vi "Test adler32.vi"() -> (3 "All Passed?":bool)   [LabVIEW 2022 SP3]
uses:
  Source/LabVIEW-Hashlib.lvlib
panel:
  out "ADLER-32 out":T1(array[cluster]) {"ADLER-32" format="%08x"}
  in  "ADLER-32 Tests":T2(array[cluster])=[{"Name"="ADLER-32/Empty", "ADLER-32"=1, "Data"="", "Initial"=1}, {"Name"="ADLER-32/Short", "ADLER-32"=300286872, "Data"="Wikipedia", "Initial"=1}, {"Name"="ADLER-32/Long", "ADLER-32"=159591549, "Data"="abcdefghijklmnopqrstuvwxyzabcdefghijklmnopqrstuvwxyzabcdefghijklmnopqrstuvwxyzabcdefghijklmnopqrstuvwxyz", "Initial"=1}, {"Name"="ADLER-32/Concat", "ADLER-32"=645159161, "Data"="abcdefghijklmnopqrstuvwxyzabcdefghijklmnopqrstuvwxyzabcdefghijklmnopqrstuvwxyzabcdefghijklmnopqrstuvwxyz", "Initial"=159591549}] {"ADLER-32" format="%08x"; "Initial" format="%08x"}
  # "http://www.unit-conversion.info/texttools/adler-32/"
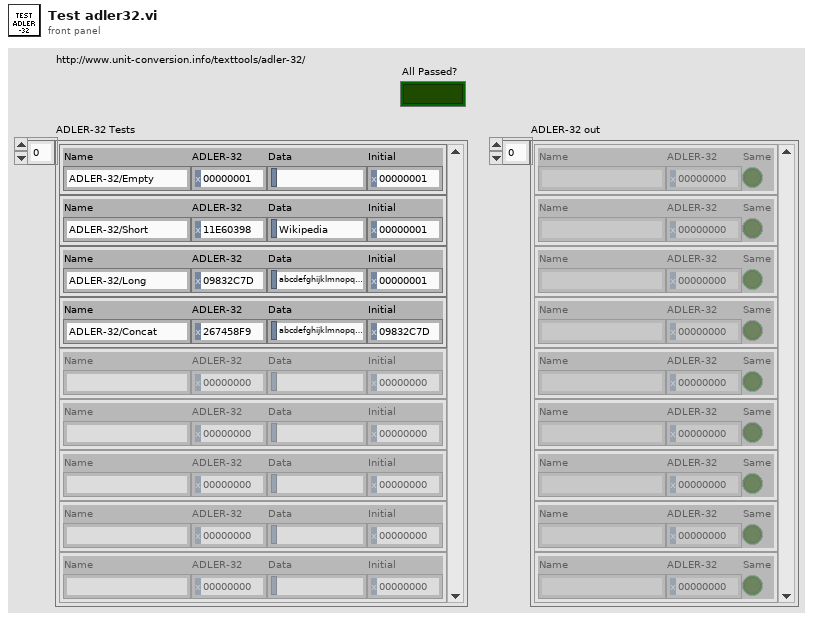
[diagram p1: front panel]
types:
  T1 = cluster{"Name":string, "ADLER-32":u32, "Same":bool}[]
  T2 = cluster{"Name":string, "ADLER-32":u32, "Data":string, "Initial":u32}[]
  T3 = cluster{"Name":string, "ADLER-32":u32, "Same":bool}
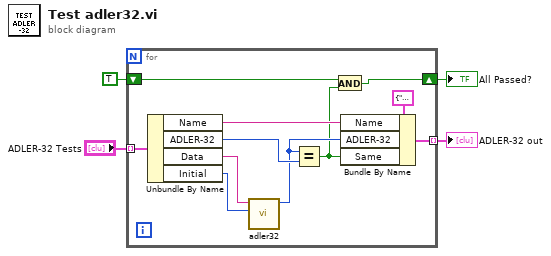
[diagram p0: block diagram]
diagram:
  n1 = for {
    tunnel: "ADLER-32 Tests" -> [w15] mode=indexing
    tunnel: [w13] -> w3 mode=indexing
    shift-right: [w8] -> w1
    shift-left: TRUE -> [w10]
    n2 = Unbundle By Name(w15) -> ("Name"=w14:string, "ADLER-32"=w12:u32, "Data"=w5:string, "Initial"=w7:u32)
    n3 = call "adler32.vi"("ADLER-32 in (1)"=w7, "Data in"=w5) -> ("ADLER-32 out"=w11:u32)  [unwired: 9 in]
    n4 = Equal?(x=w11, y=w12) -> (x = y?=w9:bool)
    n5 = And(x=w10, y=w9) -> (x .and. y?=w8:bool)
    n6 = Bundle By Name(cluster=T3 {"Name"="", "ADLER-32"=0, "Same"=FALSE} ("CRC-16"), "Name"=w14, "ADLER-32"=w11, "Same"=w9) -> (w13:T3)
  }
  "ADLER-32 out" <- w3
  "All Passed?" <- w1
